vi "StackerStateMachine.vi"(0 "HMI to Control":T7, 1 "Arm Arrived":bool, 2 "StackClampState":T1, 5 "SensorInputData":T6, 7 "Intake Wheel State":T3, 9 "Tusk State":T4, 11 "error in":errorcluster) -> (4 "HMI to Control  Out":T7={"RightDriveValue"=0.0, "LeftDriveValue"=0.0, "Arm Manual "=0.0, "Stacker Manual "=0.0, "Claw Manual "=0.0, "ClawSlightOpenNumber"=0, "Intake Value "=0.0, "Arm States"=enum."4 Tote", "Claw States"=enum."Claw Manual ", "Intake Man. or Sense"=enum."Sensing", "Stacker in Manual?"=FALSE, "Drop Stack? "=FALSE, "Tusk Up Request"=FALSE, "Tusk Down Request"=FALSE, "Inver. Wheels  In Request"=FALSE, "Inverse. Wheels Out Request "=FALSE, "Get Out of Manual Control"=FALSE, "Exit Score State"=FALSE, "DriveStraight Help?"=FALSE, "Stacker Shut Off No."=0, "Stacker Need Off?"=FALSE, "Collecting?"=FALSE, "Go to Hover"=FALSE, "Stack Clamp Lock "=FALSE, "Stack Clamp Unlock "=FALSE, "Claw Intake Value "=0.0, "Stack Clamp Lock No. "=0, "Steal Can (ruin their day?)"=FALSE, "Retract (have mercy?)"=FALSE, "Can Grab No. "=0, "Wench Value to Control "=0.0}, 6 "SensorInputData out":T6, 8 "# of Totes Out":i32, 10 "Stacker State to Index":T5=enum."Hold", 12 "Tusk State to Actuate":T4, 13 "StackClampState to Actuate":T1, 14 "Intake Wheel State to Actuate":T3, 15 "error out":errorcluster)   [LabVIEW 2014]
uses:
  Typedefs/StackerStates.ctl
  Typedefs/HMI_to_Control.ctl
  Typedefs/Arm States.ctl
  Typedefs/ClawStates.ctl
  Typedefs/IntakeWheelSenseOrManual.ctl
  Typedefs/SensorInputData.ctl
  Typedefs/TuskStates.ctl
  Typedefs/IntakeWheelStates.ctl
  Typedefs/StackClampStates.ctl
  Typedefs/ClawStateMachine.ctl
  Gensubs/Bert_or_Ernie.vi
panel:
  in  "Ernie Needed Ranges":T2={"5 on ground upper range"=196.0, "5 on ground lower range"=182.0, "6 on ground upper range"=220.0, "6 on ground on lower range"=200.0, "Hold 4 Up Limit"=17.2, "Hold 4 Low Limit "=10.0, "Hold 5 Up Limit"=15.7, "Hold 5 Low Limit"=10.0, "Get Tote Upper Ok Range "=0.6, "Get Tote Lower Ok Range"=-2.0, "Drop Stack Upper Ok Range"=0.3, "Drop Stack Lower Ok Range"=-0.5, "6 Tote Cal Upper Range"=90.0, "6 Tote Cal Lower Range"=85.0, "5 Tote Cal Upper Range "=90.0, "5 Tote Cal Lower Range "=76.0, "Stacker on Ground Bottom #"=1.5, "Hold 4 on Ground Upper Range  "=172.0, "4 on ground U.R"=174.0, "4 on ground L.R"=165.0} {"4 on ground L.R" format="%#_13g"; "4 on ground U.R" format="%#_13g"; "6 Tote Cal Upper Range" format="%#_13g"}
  in  "Bert Needed Ranges":T2={"5 on ground upper range"=193.0, "5 on ground lower range"=176.0, "6 on ground upper range"=212.0, "6 on ground on lower range"=204.0, "Hold 4 Up Limit"=21.0, "Hold 4 Low Limit "=10.0, "Hold 5 Up Limit"=18.5, "Hold 5 Low Limit"=10.5, "Get Tote Upper Ok Range "=0.7, "Get Tote Lower Ok Range"=-2.0, "Drop Stack Upper Ok Range"=0.5, "Drop Stack Lower Ok Range"=-0.5, "6 Tote Cal Upper Range"=90.0, "6 Tote Cal Lower Range"=85.0, "5 Tote Cal Upper Range "=90.0, "5 Tote Cal Lower Range "=54.0, "Stacker on Ground Bottom #"=1.5, "Hold 4 on Ground Upper Range  "=172.0, "4 on ground U.R"=174.0, "4 on ground L.R"=157.0} {"4 on ground L.R" format="%#_13g"; "4 on ground U.R" format="%#_13g"; "6 Tote Cal Upper Range" format="%#_13g"}
  out "Stacker State Out":T5=enum."Hold"
  out "Stacker State In":T5
  # "When to \nadvance\nto \nother ranges\n\nHas to match\nsetpoints\nin stacker\nsub vi"
  # "4 Bar checks\nmust be \nin line with\ncals\nin 4 bar\nsub vi"
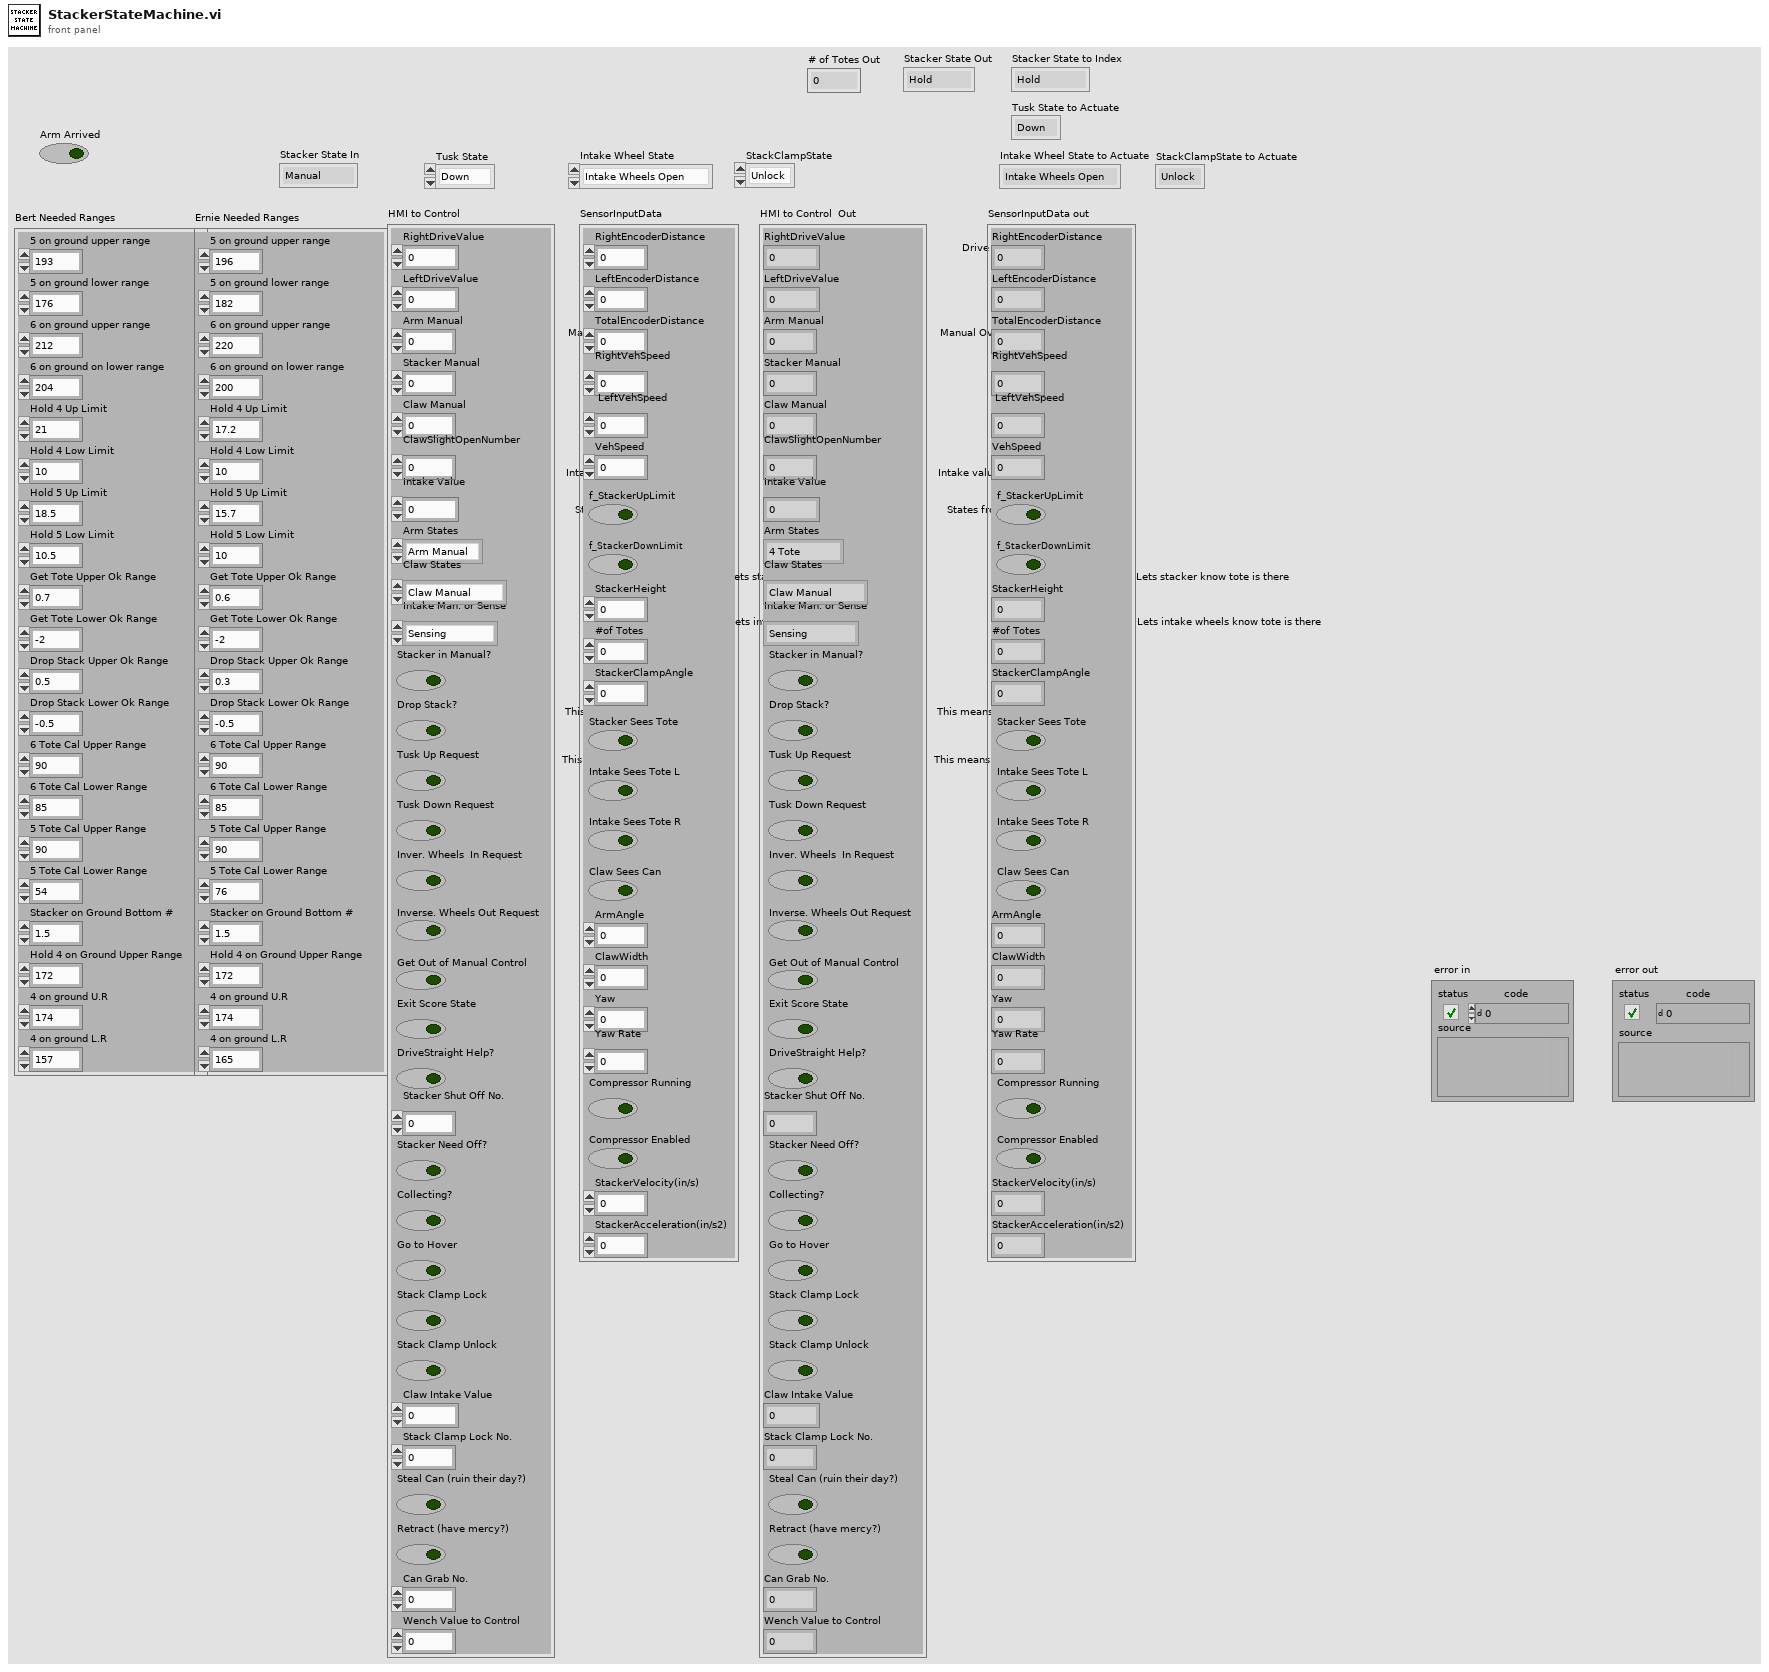
[diagram p1: front panel]
types:
  T1 = typedef "StackClampStates.ctl" = enum16{"Unlock", "Lock"}
  T2 = cluster{"5 on ground upper range":dbl, "5 on ground lower range":dbl, "6 on ground upper range":dbl, "6 on ground on lower range":dbl, "Hold 4 Up Limit":dbl, "Hold 4 Low Limit ":dbl, "Hold 5 Up Limit":dbl, "Hold 5 Low Limit":dbl, "Get Tote Upper Ok Range ":dbl, "Get Tote Lower Ok Range":dbl, "Drop Stack Upper Ok Range":dbl, "Drop Stack Lower Ok Range":dbl, "6 Tote Cal Upper Range":dbl, "6 Tote Cal Lower Range":dbl, "5 Tote Cal Upper Range ":dbl, "5 Tote Cal Lower Range ":dbl, "Stacker on Ground Bottom #":dbl, "Hold 4 on Ground Upper Range  ":dbl, "4 on ground U.R":dbl, "4 on ground L.R":dbl}
  T3 = typedef "IntakeWheelStates.ctl" = enum16{"Intake Wheels Open", "Intake Wheels Closed", "Decide off of Input", "Delay before Close", "Operator Request"}
  T4 = typedef "TuskStates.ctl" = enum16{"Down", "Up"}
  T5 = typedef "StackerStates.ctl" = enum16{"Manual ", "Hold", "Hold5", "Hold6", "GetTote", "DropStack", "Hover", "Hover5", "Wait for Up", "DecideHold", "DownTimerPeriod", "Prep Intake for Drop", "Check Arm before 5", "Make Arm ready for 5", "Check Arm before 6", "Make Arm ready for 6", "Delay for 5", "Delay for 6"}
  T6 = typedef "SensorInputData.ctl" = cluster{"RightEncoderDistance":dbl, "LeftEncoderDistance":dbl, "TotalEncoderDistance":dbl, "RightVehSpeed":dbl, "LeftVehSpeed":dbl, "VehSpeed":dbl, "f_StackerUpLimit":bool, "f_StackerDownLimit":bool, "StackerHeight":dbl, "#of Totes":u8, "StackerClampAngle":dbl, "Stacker Sees Tote":bool, "Intake Sees Tote L":bool, "Intake Sees Tote R":bool, "Claw Sees Can":bool, "ArmAngle":dbl, "ClawWidth":dbl, "Yaw":dbl, "Yaw Rate":dbl, "Compressor Running":bool, "Compressor Enabled":bool, "StackerVelocity(in/s)":dbl, "StackerAcceleration(in/s2)":dbl}
  T7 = typedef "HMI_to_Control.ctl" = cluster{"RightDriveValue":dbl, "LeftDriveValue":dbl, "Arm Manual ":dbl, "Stacker Manual ":dbl, "Claw Manual ":dbl, "ClawSlightOpenNumber":i8, "Intake Value ":sgl, "Arm States":T8, "Claw States":T9, "Intake Man. or Sense":T10, "Stacker in Manual?":bool, "Drop Stack? ":bool, "Tusk Up Request":bool, "Tusk Down Request":bool, "Inver. Wheels  In Request":bool, "Inverse. Wheels Out Request ":bool, "Get Out of Manual Control":bool, "Exit Score State":bool, "DriveStraight Help?":bool, "Stacker Shut Off No.":i8, "Stacker Need Off?":bool, "Collecting?":bool, "Go to Hover":bool, "Stack Clamp Lock ":bool, "Stack Clamp Unlock ":bool, "Claw Intake Value ":sgl, "Stack Clamp Lock No. ":i8, "Steal Can (ruin their day?)":bool, "Retract (have mercy?)":bool, "Can Grab No. ":i8, "Wench Value to Control ":dbl}
  T8 = typedef "Arm States.ctl" = enum16{"Arm Manual ", "Ground", "Step", "1 Tote", "2 Tote", "3 Tote", "4 Tote", "5 Tote", "6 Tote", "Flip Can Arm", "Grab Can in auto", "Nudge"}
  T9 = typedef "ClawStates.ctl" = enum16{"Claw Manual ", "Claw Open", "Claw Closed", "Claw Slight Open", "Flip Can"}
  T10 = typedef "IntakeWheelSenseOrManual.ctl" = enum16{"Sensing", "Manual "}
  T11 = typedef "ClawStateMachine.ctl" = enum16{"Claw User Control", "Claw State Closed", "Claw State Slight Open"}
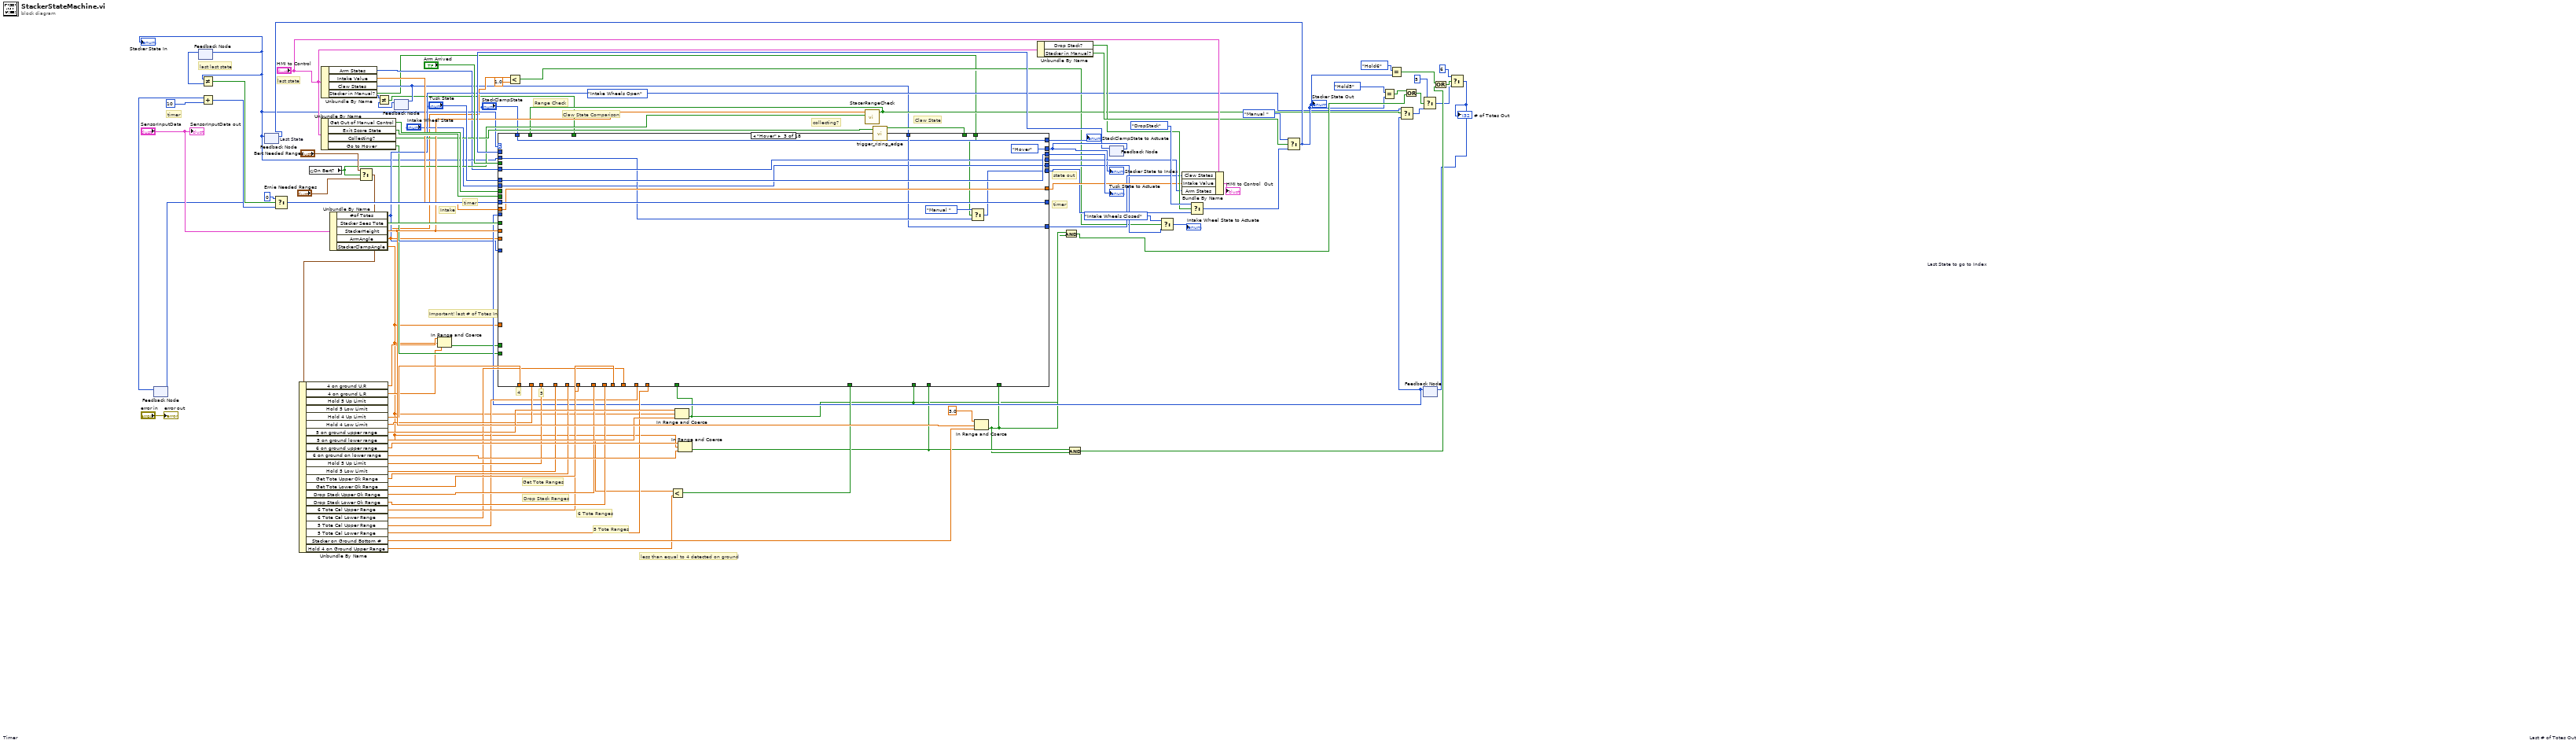
[diagram p0: block diagram]
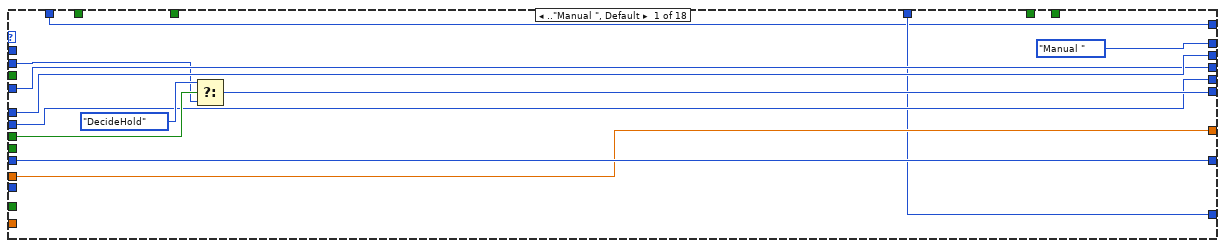
[diagram p2: hidden frame]
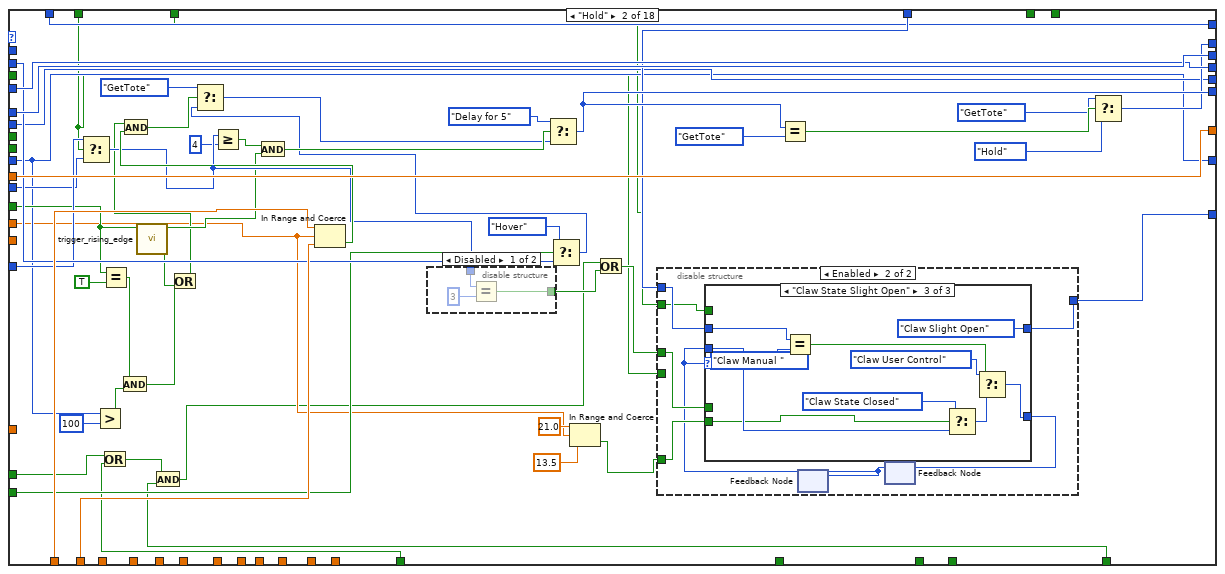
[diagram p3: hidden frame]
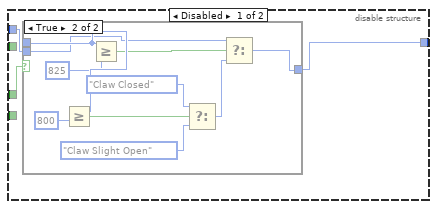
[diagram p4: hidden frame]
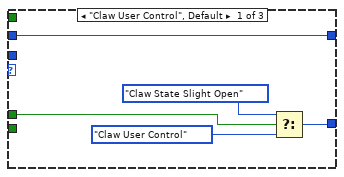
[diagram p6: hidden frame]
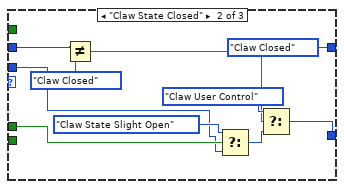
[diagram p7: hidden frame]
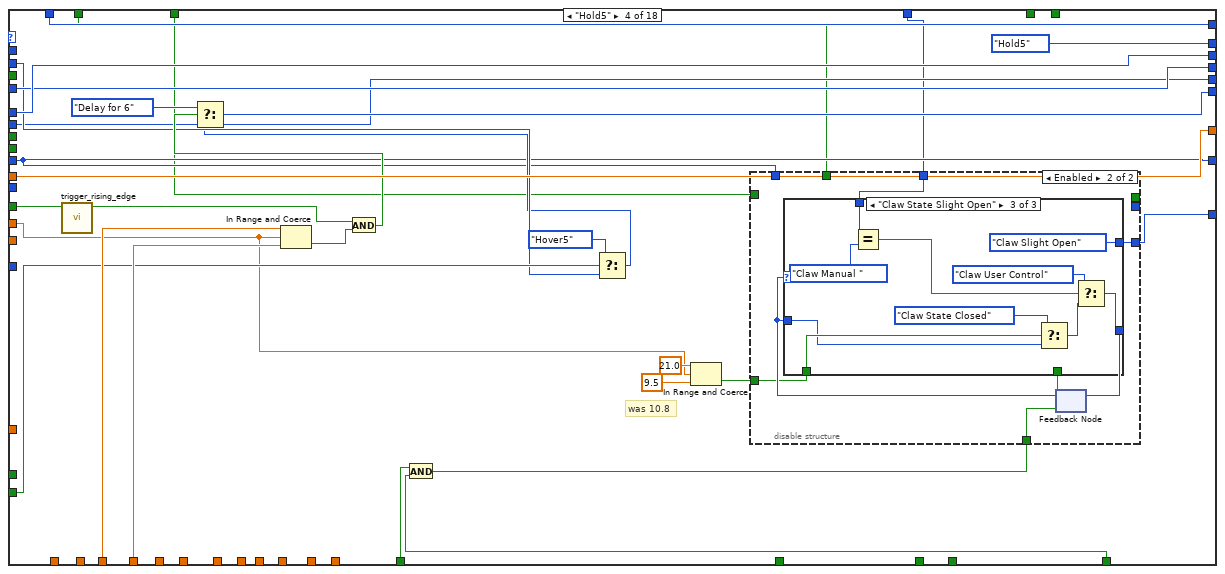
[diagram p9: hidden frame]
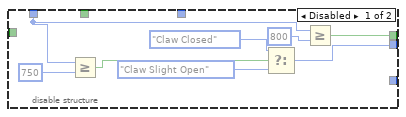
[diagram p10: hidden frame]
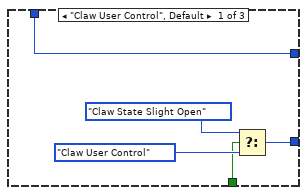
[diagram p11: hidden frame]
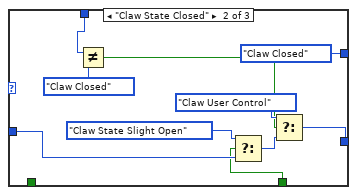
[diagram p12: hidden frame]
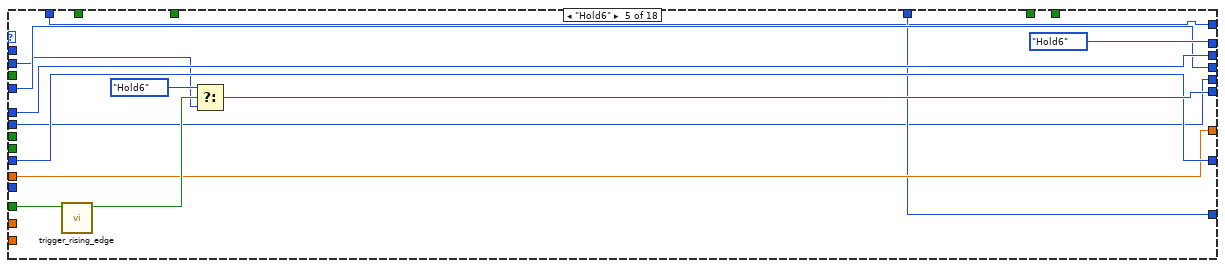
[diagram p13: hidden frame]
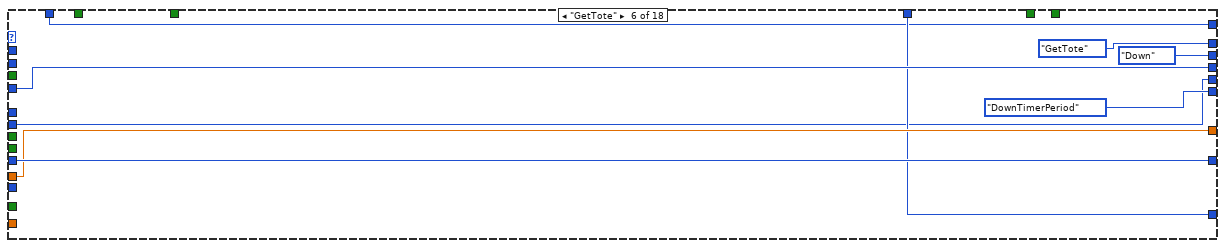
[diagram p14: hidden frame]
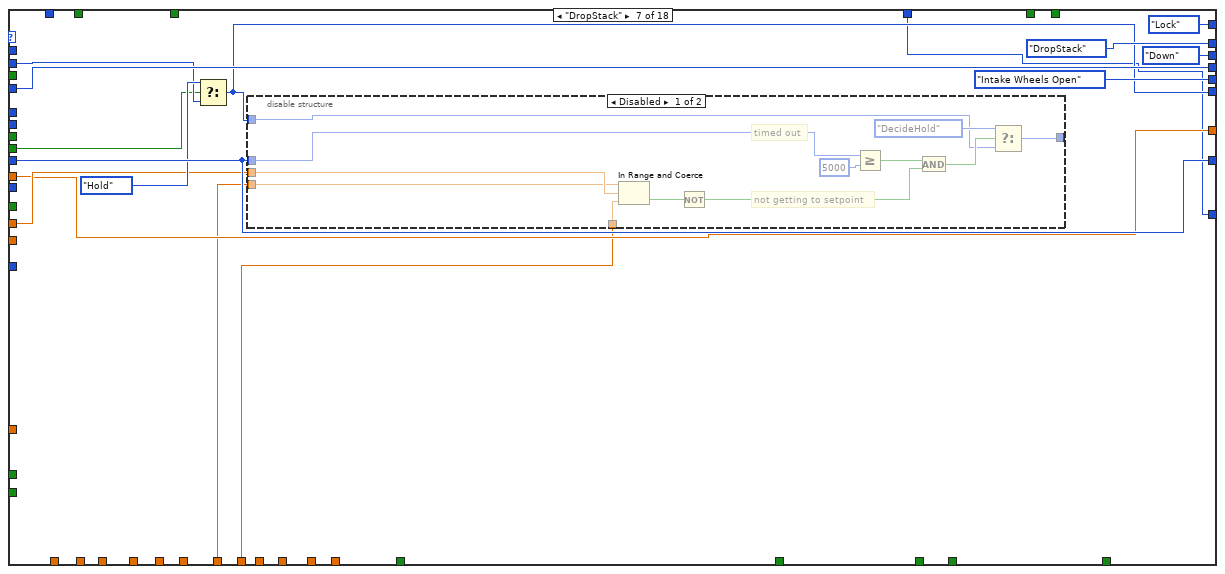
[diagram p15: hidden frame]
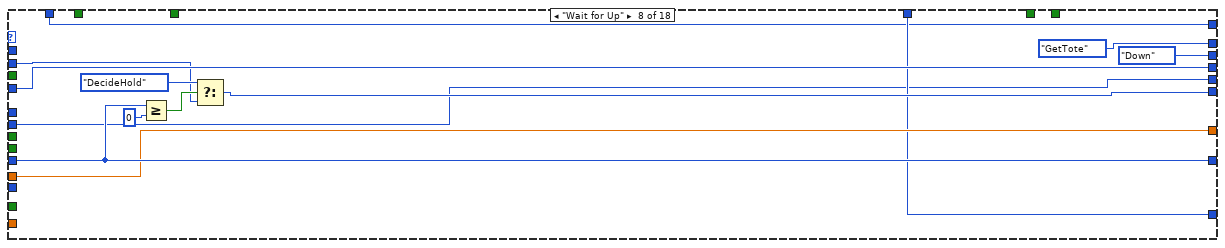
[diagram p17: hidden frame]
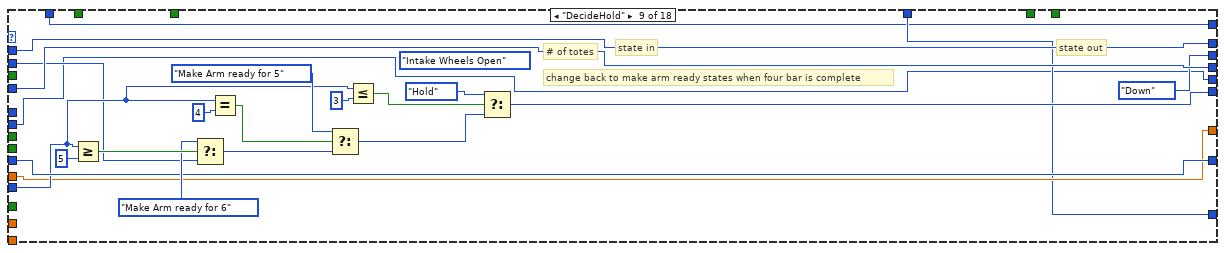
[diagram p18: hidden frame]
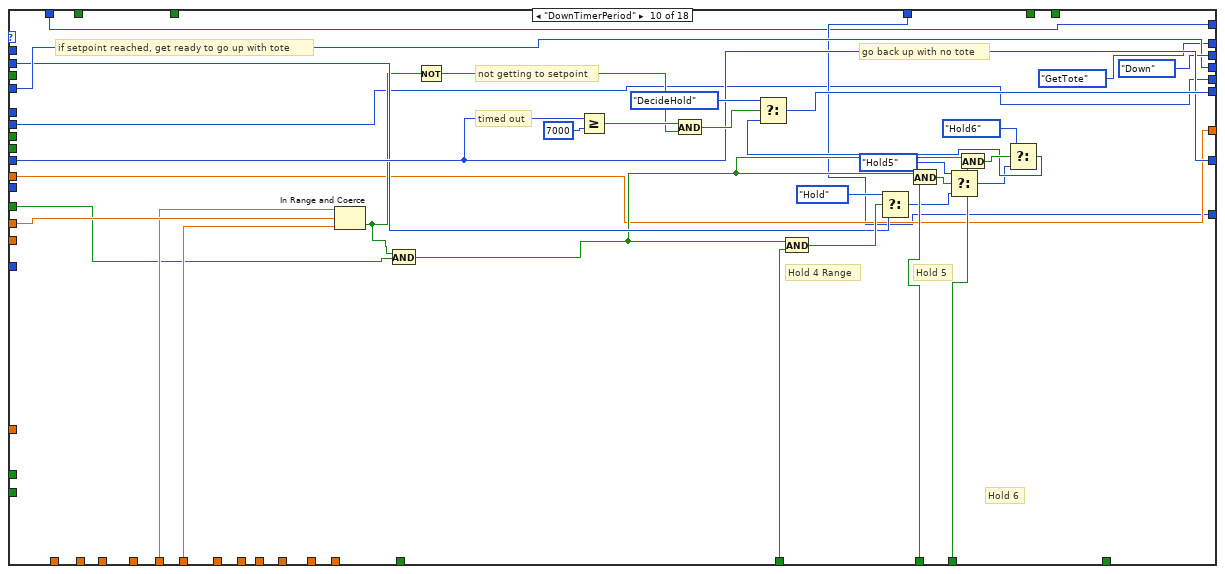
[diagram p19: hidden frame]
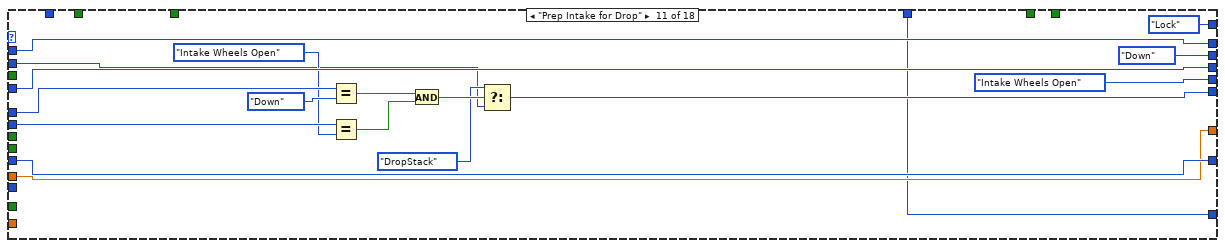
[diagram p20: hidden frame]
diagram:
  (unwired) IntakeWheelStates."Intake Wheels Open" ("y")
  # "Claw State Comparison"
  # "Range Check"
  # "Claw State"
  # "collecting?"
  # "less than equal to 4 detected on ground"
  # "5 Tote Ranges"
  # "6 Tote Ranges"
  # "Drop Stack Ranges"
  # "Get Tote Ranges"
  # "5"
  # "4"
  # "timer"
  # "state out"
  # "Important! last # of Totes In"
  # "Intake"
  # "timer"
  # "last state"
  # "last last state"
  # "timer"
  n1 = feedback #1 "Timer"() -> (w76:u32)  [unwired: 1 in]
  n2 = feedback #2() -> (w74:T5)  [unwired: 1 in]
  n3 = Add(x=w76, y=u32 10) -> (x+y=w92:u32)
  n4 = feedback #3 "Last State"() -> (w20:T5)  [unwired: 1 in]
  "Stacker State In" <- w20
  n5 = feedback-in #2(w20) -> ()
  n6 = Not Equal?(x=w20, y=w74) -> (x != y?=w91:bool)
  n7 = Select(t=u32 0, s=w91, f=w92) -> (s? t:f=w73:u32)
  n8 = global read "Bert_or_Ernie.vi" "On Bert?"() -> (w26:bool)
  n9 = Unbundle By Name("HMI to Control") -> ("Get Out of Manual Control"=w80:bool, "Exit Score State"=w79:bool, "Collecting?"=w30:bool, "Go to Hover"=w27:bool)
  n10 = Unbundle By Name("HMI to Control") -> ("Arm States"=w17:T8, "Intake Value"=w70:sgl, "Claw States"=w10:T9, "Stacker in Manual?"=w1:bool)
  n11 = Unbundle By Name("SensorInputData") -> ("#of Totes"=w28:u8, "Stacker Sees Tote"=w72:bool, "StackerHeight"=w68:dbl, "ArmAngle"=w13:dbl, "StackerClampAngle"=w3:dbl)
  n12 = Select(t="Bert Needed Ranges", s=w26, f="Ernie Needed Ranges") -> (s? t:f=w49:T2)
  n13 = Unbundle By Name(w49) -> ("4 on ground U.R"=w5:dbl, "4 on ground L.R"=w4:dbl, "Hold 4 Up Limit"=w62:dbl, "Hold 4 Low Limit"=w61:dbl, "5 on ground upper range"=w67:dbl, "5 on ground lower range"=w65:dbl, "6 on ground upper range"=w64:dbl, "6 on ground on lower range"=w63:dbl, "Hold 5 Up Limit"=w60:dbl, "Hold 5 Low Limit"=w59:dbl, "Get Tote Upper Ok Range"=w58:dbl, "Get Tote Lower Ok Range"=w57:dbl, "Drop Stack Upper Ok Range"=w56:dbl, "Drop Stack Lower Ok Range"=w55:dbl, "6 Tote Cal Upper Range"=w54:dbl, "6 Tote Cal Lower Range"=w53:dbl, "5 Tote Cal Upper Range"=w52:dbl, "5 Tote Cal Lower Range"=w51:dbl, "Stacker on Ground Bottom #"=w34:dbl, "Hold 4 on Ground Upper Range"=w33:dbl)  [unwired: 2 out]
  n14 = feedback-in #4(w10) -> ()
  n15 = feedback #4() -> (w9:T9)  [unwired: 1 in]
  n16 = Not Equal?(x=w10, y=w9) -> (x != y?=w8:bool)
  n17 = In Range and Coerce(upper limit=w5, x=w3, lower limit=w4) -> (In Range?=w7:bool)  [unwired: 1 out]
  n18 = Less?(x=w13, y=1.0) -> (x < y?=w11:bool)
  n19 = Less?(x=w3, y=w33) -> (x < y?=w32:bool)
  n20 = In Range and Coerce(upper limit=w67, x=w3, lower limit=w65) -> (In Range?=w2:bool)  [unwired: 1 out]
  n21 = In Range and Coerce(upper limit=w64, x=w3, lower limit=w63) -> (In Range?=w25:bool)  [unwired: 1 out]
  n22 = call "StacerRangeCheck.vi"("On Bert?"=w26, "Stacker"=w68) -> ("In ok range to count?"=w24:bool)  [unwired: 9 in]
  n23 = call "trigger_rising_edge.vi"("input"=w30) -> ("rising"=w22:bool)  [unwired: 10 in]
  n24 = In Range and Coerce(upper limit=3.0, x=w68, lower limit=w34) -> (In Range?=w6:bool)  [unwired: 1 out]
  n25 = Unbundle By Name("HMI to Control") -> ("Drop Stack?"=w85:bool, "Stacker in Manual?"=w89:bool)
  n26 = And(x=w6, y=w2) -> (x .and. y?=w46:bool)
  n27 = And(x=w25, y=w6) -> (x .and. y?=w37:bool)
  n28 = feedback #5 "Last State to go to Index"() -> (w75:T5)  [unwired: 1 in]
  n29 = feedback #6 "Last # of Totes Out"() -> (w29:i32)  [unwired: 1 in]
  n30 = case shown="\"Hover\"" w20 {
    tunnel: [w106 w150 w215 w251 w303 StackerStates."DownTimerPeriod" ("Enum") w322 w350 w365 w404 w415 w432 w451 w473 w487 w513 w531 w555] -> w31
    tunnel: w72 -> [_ w130 _ w250 w300 _ _ _ _ w390 _ _ _ _ _ _ _ _]
    tunnel: w73 -> [w105 w127 w222 w236 w302 w313 w325 w349 w364 w402 w413 w431 w456 w471 w497 w512 w532 w546]
    tunnel: [w105 w127 w222 w236 w302 w313 w325 w349 w364 w402 w413 w431 w456 w471 w497 w512 w532 w546] -> w78
    tunnel: [StackerStates."Manual " ("State In 2") w146 StackerStates."Hover" ("t") StackerStates."Hold5" ("Enum") StackerStates."Hold6" ("Enum") StackerStates."GetTote" ("State In 2") StackerStates."DropStack" ("State In 2") StackerStates."GetTote" ("State In 2") w363 StackerStates."GetTote" ("State In 2") w414 StackerStates."GetTote" ("State In 2") w446 StackerStates."GetTote" ("State In 2") w482 w520 w528 StackerStates."Hover" ("t")] -> w77
    tunnel: "Tusk State" -> [w104 w160 w220 w252 w301 _ _ _ _ _ w423 _ _ _ _ w519 w527 w552]
    tunnel: "Intake Wheel State" -> [w103 w132 w212 w234 w292 w305 _ w341 w354 w376 w421 _ _ _ _ w517 w525 w539]
    tunnel: [w104 w160 w220 w252 w301 TuskStates."Down" ("Tusk State") TuskStates."Down" ("Tusk State") TuskStates."Down" ("Tusk State") TuskStates."Down" ("Tusk State") TuskStates."Down" ("Tusk State") TuskStates."Down" ("Tusk State") TuskStates."Down" ("Tusk State") TuskStates."Down" ("Tusk State") TuskStates."Down" ("Tusk State") TuskStates."Down" ("Tusk State") w519 w527 w552] -> w83
    tunnel: [w103 w132 w212 w234 w292 w305 IntakeWheelStates."Intake Wheels Open" ("Intake Wheel States") w341 w354 w376 IntakeWheelStates."Intake Wheels Open" ("Intake Wheel States") IntakeWheelStates."Intake Wheels Closed" ("Intake Wheel States") IntakeWheelStates."Intake Wheels Closed" ("Intake Wheel States") IntakeWheelStates."Intake Wheels Closed" ("Intake Wheel States") IntakeWheelStates."Intake Wheels Closed" ("Intake Wheel States") w517 w525 w539] -> w15
    tunnel: w75 -> [_ _ _ _ _ _ _ _ w363 _ w414 _ w447 _ w483 w520 w528 _]
    tunnel: w17 -> [w102 w159 w219 w247 w296 w309 w327 w346 w362 w400 w426 w434 w461 w474 w494 w518 w526 w553]
    tunnel: [w102 w159 w219 w247 w296 w309 w327 w346 w362 w400 w426 w430 w459 w470 w498 w518 w526 w553] -> w82
    tunnel: "Arm Arrived" -> [_ _ _ _ _ _ _ _ _ _ _ _ _ _ _ _ _ _]
    tunnel: w80 -> [w108 _ _ _ _ _ _ _ _ _ _ _ _ _ _ _ _ _]
    tunnel: w68 -> [_ w119 _ w225 _ _ w323 _ _ w399 _ _ _ _ _ w508 w529 _]
    tunnel: w79 -> [_ _ _ _ _ _ w315 _ _ _ _ _ _ _ _ _ _ _]
    tunnel: w29 -> [_ w137 _ _ _ _ _ _ w360 _ _ _ _ _ _ _ _ _]
    tunnel: [w101 w158 w218 w249 w298 w308 w321 w344 w357 w382 w412 w429 w455 w467 w493 w516 w530 w554] -> w71
    tunnel: w70 -> [w101 w158 w218 w249 w298 w308 w321 w344 w357 w382 w412 w429 w455 w467 w493 w516 w530 w554]
    tunnel: w13 -> [_ _ _ _ _ _ _ _ _ _ _ _ w454 _ w492 _ _ _]
    tunnel: w20 -> [w100 w143 w216 w238 w295 _ w320 w345 w358 w393 w411 _ w452 _ w490 w507 w533 w556]
    tunnel: w62 -> [_ w152 _ _ _ _ _ _ _ _ _ _ _ _ _ w506 _ _]
    tunnel: w61 -> [_ w151 _ _ _ _ _ _ _ _ _ _ _ _ _ w505 _ _]
    tunnel: w60 -> [_ _ _ w245 _ _ _ _ _ _ _ _ _ _ _ _ w524 _]
    tunnel: w59 -> [_ _ _ w244 _ _ _ _ _ _ _ _ _ _ _ _ w523 _]
    tunnel: w58 -> [_ _ _ _ _ _ _ _ _ w397 _ _ _ _ _ _ _ _]
    tunnel: w57 -> [_ _ _ _ _ _ _ _ _ w396 _ _ _ _ _ _ _ _]
    tunnel: w56 -> [_ _ _ _ _ _ w319 _ _ _ _ _ _ _ _ _ _ _]
    tunnel: w55 -> [_ _ _ _ _ _ w318 _ _ _ _ _ _ _ _ _ _ _]
    tunnel: w54 -> [_ _ _ _ _ _ _ _ _ _ _ _ w445 _ w489 _ _ _]
    tunnel: w53 -> [_ _ _ _ _ _ _ _ _ _ _ _ w444 _ w488 _ _ _]
    tunnel: w52 -> [_ _ _ _ _ _ _ _ _ _ _ _ _ _ _ _ _ _]
    tunnel: w51 -> [_ _ _ _ _ _ _ _ _ _ _ _ _ _ _ _ _ _]
    tunnel: w32 -> [_ _ _ _ _ _ _ _ _ w395 _ _ _ _ _ _ _ _]
    tunnel: w2 -> [_ _ _ _ _ _ _ _ _ w384 _ _ _ _ _ _ _ _]
    tunnel: w25 -> [_ _ _ _ _ _ _ _ _ w385 _ _ _ _ _ _ _ _]
    tunnel: w22 -> [_ _ _ _ _ _ _ _ _ _ _ _ _ _ _ _ _ w557]
    tunnel: w28 -> [_ w138 _ _ _ _ _ _ _ _ _ _ _ _ _ _ _ _]
    tunnel: w27 -> [_ w141 _ w239 _ _ _ _ _ _ _ _ _ _ _ _ _ _]
    tunnel: [w99 w139 w214 w223 w294 w307 w316 w343 w356 w378 w410 w428 w443 w466 w481 w504 w522 w541] -> w21
    tunnel: w10 -> [w99 w140 w214 w231 w294 w307 w316 w343 w356 w378 w410 w428 w443 w466 w481 w504 w522 w542]
    tunnel: w24 -> [_ w122 _ w233 _ _ _ _ _ _ _ _ _ _ _ _ _ _]
    tunnel: "StackClampState" -> [w98 w133 w213 w235 w293 w306 _ w342 w355 w377 _ w427 w442 w465 w480 w503 w521 w540]
    tunnel: [w98 w133 w213 w235 w293 w306 StackClampStates."Lock" ("StackClampState") w342 w355 w377 StackClampStates."Lock" ("StackClampState") w427 w442 w465 w480 w503 w521 w540] -> w18
    tunnel: w8 -> [_ w123 _ w232 _ _ _ _ _ _ _ _ _ _ _ _ _ _]
    tunnel: w7 -> [_ w113 _ _ _ _ _ _ _ _ _ _ _ _ _ _ _ _]
    tunnel: w6 -> [_ w118 _ w230 _ _ _ _ _ _ _ _ _ _ _ _ _ _]
    tunnel: w3 -> [_ _ _ _ _ _ _ _ _ _ _ _ _ _ _ _ _ _]
    tunnel: w2 -> [_ w111 _ w224 _ _ _ _ _ _ _ _ _ _ _ _ _ _]
    tunnel: w1 -> [_ _ w211 _ _ _ _ _ _ _ _ _ _ _ _ _ _ _]
    frame .."Manual ", Default {
      n31 = Select(t=StackerStates."DecideHold" ("State In 2"), s=w108, f=w100) -> (s? t:f=w106:T5)
    }
    frame "Hold" {
      n32 = Select(t=w138, s=w122, f=w137) -> (s? t:f=w136:i32)
      n33 = Greater?(x=w127, y=u32 100) -> (0:w114:bool)
      n34 = Or(x=w113, y=w111) -> (x .or. y?=w112:bool)
      n35 = Equal?(x=w130, y=TRUE) -> (x = y?=w128:bool)
      n36 = And(x=w128, y=w114) -> (x .and. y?=w125:bool)
      n37 = call "trigger_rising_edge.vi"("input"=w130) -> ("rising"=w131:bool)  [unwired: 10 in]
      n38 = And(x=w112, y=w118) -> (x .and. y?=w115:bool)
      n39 = Or(x=w125, y=w131) -> (x .or. y?=w124:bool)
      n40 = Greater Or Equal?(x=w136, y=u8 4) -> (x >= y?=w117:bool)
      n41 = And(x=w117, y=w131) -> (x .and. y?=w157:bool)
      n42 = In Range and Coerce(upper limit=w152, x=w119, lower limit=w151) -> (In Range?=w155:bool)  [unwired: 1 out]
      n43 = And(x=w124, y=w155) -> (x .and. y?=w154:bool)
      n44 = disable-structure shown="Disabled" {
        disable-tunnel: w136 -> [w210 _]
        disable-tunnel: [w209 _] -> w135
        frame Disabled {
          n45 = Equal?(x=w210, y=3) -> (x = y?=w209:bool)
        }
        frame Enabled {
        }
      }
      n46 = Select(t=StackerStates."Hover" ("y"), s=w141, f=w143) -> (s? t:f=w142:T5)
      n47 = Select(t=StackerStates."GetTote" ("State In 2"), s=w154, f=w142) -> (s? t:f=w156:T5)
      n48 = Select(t=StackerStates."Delay for 5" ("State In 2"), s=w157, f=w156) -> (s? t:f=w150:T5)
      n49 = In Range and Coerce(upper limit=21.0, x=w119, lower limit=13.5) -> (In Range?=w110:bool)  [unwired: 1 out]
      n50 = Or(x=w115, y=w135) -> (x .or. y?=w134:bool)
      n51 = disable-structure shown="Enabled" {
        disable-tunnel: w140 -> [w164 w182]
        disable-tunnel: [w163 w181] -> w139
        disable-tunnel: w134 -> [w162 w180]
        disable-tunnel: w123 -> [_ w177]
        disable-tunnel: w122 -> [_ _]
        disable-tunnel: w110 -> [_ w178]
        frame Disabled {
          n52 = case shown="True" w162 {
            tunnel: w164 -> [w165 w167]
            tunnel: _ -> [_ w171]
            tunnel: [w165 w166] -> w163
            frame False {
            }
            frame True {
              n53 = Greater Or Equal?(x=w171, y=u32 800) -> (x >= y?=w172:bool)
              n54 = Greater Or Equal?(x=w171, y=u32 825) -> (x >= y?=w169:bool)
              n55 = Select(t=ClawStates."Claw Closed" ("Claw States"), s=w172, f=ClawStates."Claw Slight Open" ("Claw States")) -> (s? t:f=w168:T9)
              n56 = Select(t=w167, s=w169, f=w168) -> (s? t:f=w166:T9)
            }
          }
        }
        frame Enabled {
          n57 = feedback #7() -> ()  [unwired: 2 in]
          n58 = feedback #8() -> (w176:T11)  [unwired: 1 in]
          n59 = case shown="\"Claw State Slight Open\"" w176 {
            tunnel: w182 -> [w187 w190 w203]
            tunnel: [w187 ClawStates."Claw Closed" ("Claw States") ClawStates."Claw Slight Open" ("Claw States")] -> w181
            tunnel: w180 -> [w185 w193 _]
            tunnel: [w183 w191 w198] -> w179
            tunnel: w178 -> [_ _ w204]
            tunnel: w176 -> [_ w192 w206]
            tunnel: w177 -> [_ _ _]
            frame "Claw User Control", Default {
              n60 = Select(t=ClawStateMachine."Claw State Slight Open", s=w185, f=ClawStateMachine."Claw User Control") -> (s? t:f=w183:T11)
            }
            frame "Claw State Closed" {
              n61 = Not Equal?(x=w190, y=ClawStates."Claw Closed") -> (x != y?=w188:bool)
              n62 = Select(t=ClawStateMachine."Claw State Slight Open", s=w193, f=w192) -> (s? t:f=w194:T11)
              n63 = Select(t=ClawStateMachine."Claw User Control", s=w188, f=w194) -> (s? t:f=w191:T11)
            }
            frame "Claw State Slight Open" {
              n64 = Equal?(x=w203, y=ClawStates."Claw Manual ") -> (x = y?=w199:bool)
              n65 = Select(t=ClawStateMachine."Claw State Closed", s=w204, f=w206) -> (s? t:f=w201:T11)
              n66 = Select(t=ClawStateMachine."Claw User Control", s=w199, f=w201) -> (s? t:f=w198:T11)
            }
          }
          n67 = feedback-in #7(w176) -> ()
          n68 = feedback-in #8(w179) -> ()
        }
      }
      n69 = Equal?(x=w150, y=StackerStates."GetTote") -> (x = y?=w148:bool)
      n70 = Select(t=StackerStates."GetTote" ("y"), s=w148, f=StackerStates."Hold" ("State In 2")) -> (s? t:f=w146:T5)
    }
    frame "Hover" {
      n71 = Select(t=StackerStates."Manual ", s=w211, f=w216) -> (s? t:f=w215:T5)
    }
    frame "Hold5" {
      # "was 10.8"
      n72 = call "trigger_rising_edge.vi"("input"=w250) -> ("rising"=w242:bool)  [unwired: 10 in]
      n73 = In Range and Coerce(upper limit=w245, x=w225, lower limit=w244) -> (In Range?=w243:bool)  [unwired: 1 out]
      n74 = And(x=w242, y=w243) -> (x .and. y?=w241:bool)
      n75 = And(x=w224, y=w230) -> (x .and. y?=w229:bool)
      n76 = Select(t=StackerStates."Hover5" ("y"), s=w239, f=w238) -> (s? t:f=w237:T5)
      n77 = Select(t=StackerStates."Delay for 6" ("Enum"), s=w241, f=w237) -> (s? t:f=w251:T5)
      n78 = In Range and Coerce(upper limit=21.0, x=w225, lower limit=9.5) -> (In Range?=w226:bool)  [unwired: 1 out]
      n79 = disable-structure shown="Enabled" {
        disable-tunnel: w236 -> [w256 _]
        disable-tunnel: [w254 _] -> _
        disable-tunnel: [w253 _] -> _
        disable-tunnel: w233 -> [_ _]
        disable-tunnel: w232 -> [_ _]
        disable-tunnel: w231 -> [_ w266]
        disable-tunnel: w229 -> [_ w265]
        disable-tunnel: w226 -> [_ w262]
        disable-tunnel: [_ w261] -> w223
        frame Disabled {
          n80 = Greater Or Equal?(x=w256, y=u32 750) -> (x >= y?=w259:bool)
          n81 = Select(t=ClawStates."Claw Closed" ("Claw States"), s=w259, f=ClawStates."Claw Slight Open") -> (s? t:f=w253:T9)
          n82 = Greater Or Equal?(x=w256, y=u32 800) -> (x >= y?=w254:bool)
        }
        frame Enabled {
          n83 = feedback #9() -> (w263:T11)  [unwired: 1 in]
          n84 = case shown="\"Claw State Slight Open\"" w263 {
            tunnel: [w267 ClawStates."Claw Closed" ("Claw States") ClawStates."Claw Slight Open" ("Claw States")] -> w261
            tunnel: [w269 w277 w282] -> w264
            tunnel: w266 -> [w267 w274 w287]
            tunnel: w265 -> [w268 w272 _]
            tunnel: w263 -> [_ w273 w288]
            tunnel: w262 -> [_ _ w289]
            frame "Claw User Control", Default {
              n85 = Select(t=ClawStateMachine."Claw State Slight Open", s=w268, f=ClawStateMachine."Claw User Control") -> (s? t:f=w269:T11)
            }
            frame "Claw State Closed" {
              n86 = Not Equal?(x=w274, y=ClawStates."Claw Closed") -> (x != y?=w275:bool)
              n87 = Select(t=ClawStateMachine."Claw State Slight Open", s=w272, f=w273) -> (s? t:f=w278:T11)
              n88 = Select(t=ClawStateMachine."Claw User Control", s=w275, f=w278) -> (s? t:f=w277:T11)
            }
            frame "Claw State Slight Open" {
              n89 = Equal?(x=w287, y=ClawStates."Claw Manual ") -> (x = y?=w284:bool)
              n90 = Select(t=ClawStateMachine."Claw State Closed", s=w289, f=w288) -> (s? t:f=w283:T11)
              n91 = Select(t=ClawStateMachine."Claw User Control", s=w284, f=w283) -> (s? t:f=w282:T11)
            }
          }
          n92 = feedback-in #9(w264) -> ()
        }
      }
    }
    frame "Hold6" {
      n93 = call "trigger_rising_edge.vi"("input"=w300) -> ("rising"=w299:bool)  [unwired: 10 in]
      n94 = Select(t=StackerStates."Hold6" ("State Out 2"), s=w299, f=w295) -> (s? t:f=w303:T5)
    }
    frame "GetTote" {
    }
    frame "DropStack" {
      n95 = Select(t=StackerStates."Hold" ("Enum"), s=w315, f=w320) -> (s? t:f=w322:T5)
      n96 = disable-structure shown="Disabled" {
        disable-tunnel: [w334 _] -> _
        disable-tunnel: w325 -> [w333 _]
        disable-tunnel: w322 -> [w332 _]
        disable-tunnel: w323 -> [w331 _]
        disable-tunnel: w319 -> [w330 _]
        disable-tunnel: w318 -> [w329 _]
        frame Disabled {
          # "not getting to setpoint"
          # "timed out"
          n97 = In Range and Coerce(upper limit=w330, x=w331, lower limit=w329) -> (In Range?=w336:bool)  [unwired: 1 out]
          n98 = Not(x=w336) -> (.not. x?=w338:bool)
          n99 = Greater Or Equal?(x=w333, y=u32 5000) -> (x >= y?=w340:bool)
          n100 = And(x=w340, y=w338) -> (x .and. y?=w339:bool)
          n101 = Select(t=StackerStates."DecideHold" ("Stacker State In 2"), s=w339, f=w332) -> (s? t:f=w334:T5)
        }
        frame Enabled {
        }
      }
    }
    frame "Wait for Up" {
      n102 = Greater Or Equal?(x=w349, y=u32 0) -> (x >= y?=w352:bool)
      n103 = Select(t=StackerStates."DecideHold" ("Stacker State In 2"), s=w352, f=w345) -> (s? t:f=w350:T5)
    }
    frame "DecideHold" {
      (unwired) IntakeWheelStates."Intake Wheels Open" ("Intake Wheel States")
      # "# of totes"
      # "change back to make arm ready states when four bar is complete"
      # "state out"
      # "state in"
      n104 = Greater Or Equal?(x=w360, y=i8 5) -> (x >= y?=w375:bool)
      n105 = Select(t=StackerStates."Make Arm ready for 6" ("State In 2"), s=w375, f=w358) -> (s? t:f=w373:T5)
      n106 = Equal?(x=w360, y=i8 4) -> (x = y?=w371:bool)
      n107 = Select(t=StackerStates."Make Arm ready for 5" ("State In 2"), s=w371, f=w373) -> (s? t:f=w368:T5)
      n108 = Less Or Equal?(x=w360, y=i8 3) -> (x <= y?=w366:bool)
      n109 = Select(t=StackerStates."Hold" ("State In 2"), s=w366, f=w368) -> (s? t:f=w365:T5)
    }
    frame "DownTimerPeriod" {
      # "Hold 5"
      # "Hold 6"
      # "Hold 4 Range"
      # "if setpoint reached, get ready to go up with tote"
      # "go back up with no tote"
      # "not getting to setpoint"
      # "timed out"
      n110 = In Range and Coerce(upper limit=w397, x=w399, lower limit=w396) -> (In Range?=w391:bool)  [unwired: 1 out]
      n111 = And(x=w391, y=w390) -> (x .and. y?=w386:bool)
      n112 = Not(x=w391) -> (.not. x?=w406:bool)
      n113 = Greater Or Equal?(x=w402, y=u32 7000) -> (x >= y?=w408:bool)
      n114 = And(x=w408, y=w406) -> (x .and. y?=w407:bool)
      n115 = And(x=w386, y=w395) -> (x .and. y?=w394:bool)
      n116 = Select(t=StackerStates."Hold", s=w394, f=w393) -> (s? t:f=w380:T5)
      n117 = And(x=w386, y=w384) -> (x .and. y?=w389:bool)
      n118 = Select(t=StackerStates."Hold5", s=w389, f=w380) -> (s? t:f=w381:T5)
      n119 = And(x=w386, y=w385) -> (x .and. y?=w387:bool)
      n120 = Select(t=StackerStates."Hold6", s=w387, f=w381) -> (s? t:f=w383:T5)
      n121 = Select(t=StackerStates."DecideHold" ("Stacker State In 2"), s=w407, f=w383) -> (s? t:f=w404:T5)
    }
    frame "Prep Intake for Drop" {
      n122 = Equal?(x=w423, y=TuskStates."Down") -> (x = y?=w419:bool)
      n123 = Equal?(x=w421, y=IntakeWheelStates."Intake Wheels Open") -> (x = y?=w418:bool)
      n124 = And(x=w419, y=w418) -> (x .and. y?=w417:bool)
      n125 = Select(t=StackerStates."DropStack" ("Enum"), s=w417, f=w411) -> (s? t:f=w415:T5)
    }
    frame "Check Arm before 5" {
      # "Arm State"
      # "Stacker State"
      # "timer"
      # "state to index"
      n126 = Equal?(x=w434, y=Arm_States."6 Tote") -> (x = y?=w437:bool)
      n127 = Select(t=w434, s=w437, f=Arm_States."6 Tote") -> (s? t:f=w430:T8)
      n128 = Select(t=StackerStates."Hold5" ("Enum"), s=w437, f=StackerStates."Make Arm ready for 5") -> (s? t:f=w432:T5)
    }
    frame "Make Arm ready for 5" {
      # "Stacker State"
      # "Arm State"
      # "timer"
      n129 = Equal?(x=w461, y=Arm_States."6 Tote") -> (x = y?=w462:bool)
      n130 = Select(t=w461, s=w462, f=Arm_States."6 Tote") -> (s? t:f=w459:T8)
      n131 = In Range and Coerce(upper limit=w445, x=w454, lower limit=w444) -> (In Range?=w453:bool)  [unwired: 1 out]
      n132 = Select(t=StackerStates."Hold5", s=w453, f=w452) -> (s? t:f=w451:T5)
      n133 = Equal?(x=StackerStates."Hold5", y=w451) -> (x = y?=w449:bool)
      n134 = Select(t=StackerStates."Hold5" ("x"), s=w449, f=w447) -> (s? t:f=w446:T5)
    }
    frame "Check Arm before 6" {
      n135 = Equal?(x=w474, y=Arm_States."6 Tote") -> (x = y?=w476:bool)
      n136 = Select(t=w474, s=w476, f=Arm_States."6 Tote") -> (s? t:f=w470:T8)
      n137 = Select(t=StackerStates."Hold6" ("Enum"), s=w476, f=StackerStates."Make Arm ready for 6") -> (s? t:f=w473:T5)
    }
    frame "Make Arm ready for 6" {
      n138 = In Range and Coerce(upper limit=w489, x=w492, lower limit=w488) -> (In Range?=w491:bool)  [unwired: 1 out]
      n139 = Equal?(x=w494, y=Arm_States."6 Tote") -> (x = y?=w500:bool)
      n140 = Select(t=w494, s=w500, f=Arm_States."6 Tote") -> (s? t:f=w498:T8)
      n141 = Select(t=StackerStates."Hold6", s=w491, f=w490) -> (s? t:f=w487:T5)
      n142 = Equal?(x=StackerStates."Hold6" ("t"), y=w487) -> (x = y?=w485:bool)
      n143 = Select(t=StackerStates."Hold6", s=w485, f=w483) -> (s? t:f=w482:T5)
    }
    frame "Delay for 5" {
      n144 = In Range and Coerce(upper limit=w506, x=w508, lower limit=w505) -> (In Range?=w509:bool)  [unwired: 1 out]
      n145 = Greater Or Equal?(x=w512, y=u32 0) -> (x >= y?=w511:bool)
      n146 = And(x=w511, y=w509) -> (x .and. y?=w510:bool)
      n147 = Select(t=StackerStates."GetTote" ("Enum"), s=w510, f=w507) -> (s? t:f=w513:T5)
    }
    frame "Delay for 6" {
      n148 = In Range and Coerce(upper limit=w524, x=w529, lower limit=w523) -> (In Range?=w538:bool)  [unwired: 1 out]
      n149 = Greater Or Equal?(x=w532, y=u32 0) -> (x >= y?=w536:bool)
      n150 = And(x=w536, y=w538) -> (x .and. y?=w537:bool)
      n151 = Select(t=StackerStates."GetTote" ("Enum"), s=w537, f=w533) -> (s? t:f=w531:T5)
    }
    frame "Hover5" {
      n152 = Greater Or Equal?(x=w546, y=u32 1000) -> (x >= y?=w544:bool)
      n153 = Greater Or Equal?(x=w546, y=u32 1050) -> (x >= y?=w543:bool)
      n154 = Select(t=ClawStates."Claw Closed" ("Claw States"), s=w544, f=ClawStates."Claw Slight Open" ("Claw States")) -> (s? t:f=w548:T9)
      n155 = Select(t=w542, s=w543, f=w548) -> (s? t:f=w541:T9)
      n156 = Select(t=StackerStates."Hold5", s=w557, f=w556) -> (s? t:f=w555:T5)
    }
  }
  "Stacker State to Index" <- w77
  "Tusk State to Actuate" <- w83
  "StackClampState to Actuate" <- w18
  n157 = feedback-in #1(w78) -> ()
  n158 = feedback-in #5(w77) -> ()
  n159 = Select(t=IntakeWheelStates."Intake Wheels Closed" ("Intake Wheel State"), s=w11, f=w15) -> (s? t:f=→"Intake Wheel State to Actuate":T3)
  n160 = Bundle By Name(cluster="HMI to Control", "Claw States"=w21, "Intake Value"=w71, "Arm States"=w82) -> (→"HMI to Control  Out":T7)
  n161 = Select(t=StackerStates."DropStack", s=w85, f=w31) -> (s? t:f=w88:T5)
  n162 = Select(t=StackerStates."Manual ", s=w89, f=w88) -> (s? t:f=w40:T5)
  "Stacker State Out" <- w40
  n163 = feedback-in #3(w40) -> ()
  n164 = Equal?(x=StackerStates."Hold5" ("y"), y=w40) -> (x = y?=w47:bool)
  n165 = Equal?(x=StackerStates."Hold6" ("y"), y=w40) -> (x = y?=w39:bool)
  n166 = Select(t=w28, s=w24, f=w29) -> (s? t:f=w43:i32)
  n167 = Or(x=w47, y=w46) -> (x .or. y?=w45:bool)
  n168 = Select(t=5, s=w45, f=w43) -> (s? t:f=w36:i32)
  n169 = Or(x=w39, y=w37) -> (x .or. y?=w38:bool)
  n170 = Select(t=6, s=w38, f=w36) -> (s? t:f=w35:i32)
  "# of Totes Out" <- w35
  n171 = feedback-in #6(w35) -> ()
  "SensorInputData out" <- "SensorInputData"
  "error out" <- "error in"
